vi "Write Dependencies.vi"(8 "error in (no error)":errorcluster, 10 "SMOs":refnum<class "SMO.lvclass">[](array[class]), 11 "Logger.Error in":refnum<class "Logger.Error.lvclass">) -> (0 "error out":errorcluster, 3 "Logger.Error out":refnum<class "Logger.Error.lvclass">)   [LabVIEW 2019, in "Logger.Error.lvclass"]
uses:
  Logger.Error.lvclass
  <vilib>/JKI/JKI SMO/SMO/SMO.lvclass
  Logger.Error.lvclass/Logger.Error.ctl
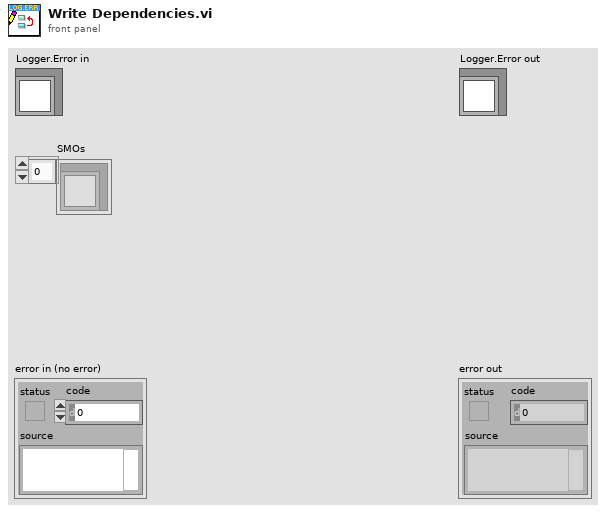
[diagram p1: front panel]
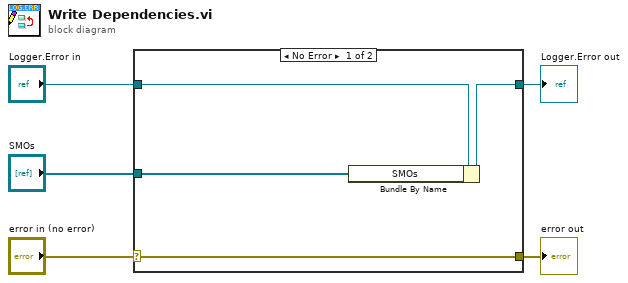
[diagram p0: block diagram]
diagram:
  n1 = case shown="No Error" "error in (no error)" {
    selector: "error in (no error)" -> [w9 w10]
    tunnel: [w9 w10] -> w4
    tunnel: [w7 w11] -> w2
    tunnel: "Logger.Error in" -> [w8 w11]
    tunnel: "SMOs" -> [w6 _]
    frame No Error {
      n2 = Bundle By Name(cluster=w8, "SMOs"=w6) -> (w7:refnum<class "Logger.Error.lvclass">)
    }
    frame Error {
    }
  }
  "error out" <- w4
  "Logger.Error out" <- w2
